vi "Read JSON Config.vi"(8 "error in (no error)":errorcluster, 10 "JSON Config":string, 11 "AbsFunc_Two Term_U8 in":refnum<class "AbsFunc_Two Term_U8.lvclass">) -> (0 "error out":errorcluster, 3 "AbsFunc_Two Term_U8 out":refnum<class "AbsFunc_Two Term_U8.lvclass">)   [LabVIEW 2021, in "AbsFunc_Two Term_U8.lvclass"]
uses:
  AbsFunc_Two Term_U8.lvclass
  C:/Program Files (x86)/National Instruments/LabVIEW 2021/vi.lib/TSA/Abstract Data Classes/Abs_Types/Type/Abs_Type.lvclass
  AbsFunc_Two Term_U8.lvclass/AbsFunc_Two Term_U8.ctl
  Abs_Types/Numeric/Abs_Numeric.lvclass
  Abs_Types/U8 Integer/Abs_U8 Integer.lvclass
  <vilib>/Utility/LVClass/Get LV Class Name.vi
  Abs_Types/Type/Abs_Type.lvclass
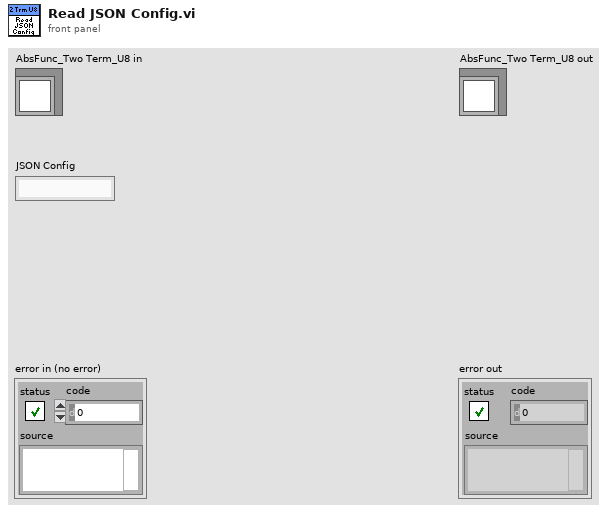
[diagram p1: front panel]
types:
  T1 = typedef "AbsFunc_Two Term_U8.lvclass/Abstract Type.ctl" = refnum<class "Abs_U8 Integer.lvclass">
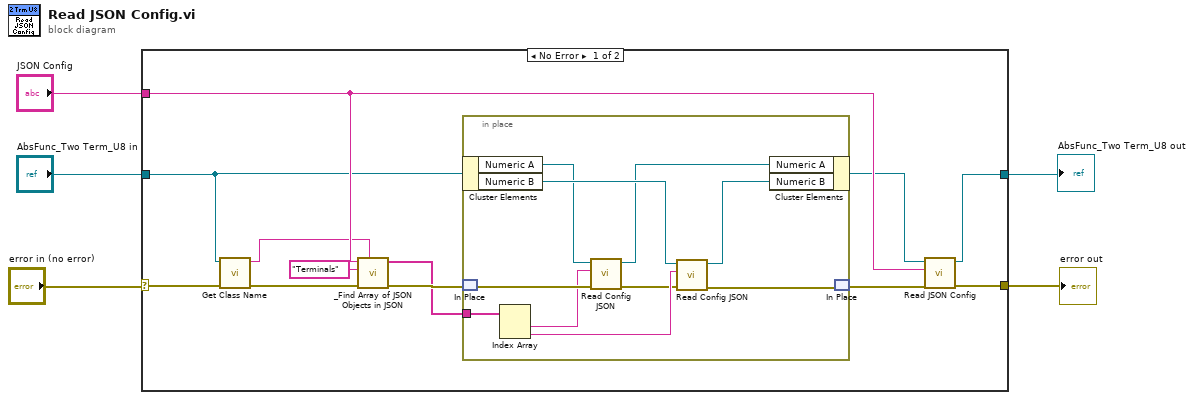
[diagram p0: block diagram]
diagram:
  n1 = case shown="No Error" "error in (no error)" {
    selector: "error in (no error)" -> [w13 w28]
    tunnel: [w17 w28] -> w4
    tunnel: [w16 w29] -> w5
    tunnel: "JSON Config" -> [w15 _]
    tunnel: "AbsFunc_Two Term_U8 in" -> [w12 w29]
    frame No Error {
      n2 = call "Get Class Name.vi"("error in (no error)"=w13, "Abs_Type in"=w12) -> ("error out"=w14:errorcluster, "class name"=w7:string)  [unwired: 8 in]
      n3 = call "_Find Array of JSON Objects in JSON.vi"("JSON Object Name"=w7, "error in (no error)"=w14, "JSON Array Name"="Terminals", "JSON Config"=w15) -> ("error out"=w11:errorcluster, "JSON Objects"=w10:string[])  [unwired: 6 in]
      n4 = in-place {
        in-place-border: w10 -> [w27]
        n5 = in-place-cluster #1(w12) -> ("Numeric A"=w19:T1, "Numeric B"=w23:refnum<class "Abs_Numeric.lvclass">)
        n6 = in-place-match #2(w11) -> (w26:errorcluster)
        n7 = Index Array(array=w27) -> (element #1=w25:string, element #2=w24:string)  [unwired: 2 in]
        n8 = call "Read Config JSON.vi"("error in (no error)"=w26, "JSON Config"=w25, "Abs_Type in"=w19) -> ("error out"=w20:errorcluster, "Abs_Type out"=w18:T1)  [unwired: 7 in]
        n9 = call "Read Config JSON.vi"("error in (no error)"=w20, "JSON Config"=w24, "Abs_Type in"=w23) -> ("error out"=w21:errorcluster, "Abs_Type out"=w22:refnum<class "Abs_Numeric.lvclass">)  [unwired: 7 in]
        n10 = in-place-cluster #1("Numeric A"=w18, "Numeric B"=w22) -> (w8:refnum<class "AbsFunc_Two Term_U8.lvclass">)
        n11 = in-place-match #2(w21) -> (w9:errorcluster)
      }
      n12 = call-parent "Read JSON Config.vi"("error in (no error)"=w9, "JSON Config"=w15, "Abs_Type in"=w8) -> ("error out"=w17:errorcluster, "Abs_Type out"=w16:refnum<class "AbsFunc_Two Term_U8.lvclass">)  [unwired: 7 in]
    }
    frame Error {
    }
  }
  "error out" <- w4
  "AbsFunc_Two Term_U8 out" <- w5
